vi "setStopServerOcc.vi"(8 "error in (no error)":errorcluster, 11 "TcpServerCmd in":refnum<class "TcpServerCmd.lvclass">) -> (0 "error out":errorcluster, 3 "TcpServerCmd out":refnum<class "TcpServerCmd.lvclass">)   [LabVIEW 2018, in "TcpServerCmd.lvclass"]
doc: "Set the stopServer occurrence to stop the runServer.vi."
uses:
  TcpServerCmd.lvclass
  home/pcortes/github/ts_labview_tcp_json/src/TcpServerBase/TcpServerBase.lvclass
  TcpServerBase/TcpServerBase.lvclass/TcpServerBase.ctl
  TcpServerBase/TcpServerBase.lvclass
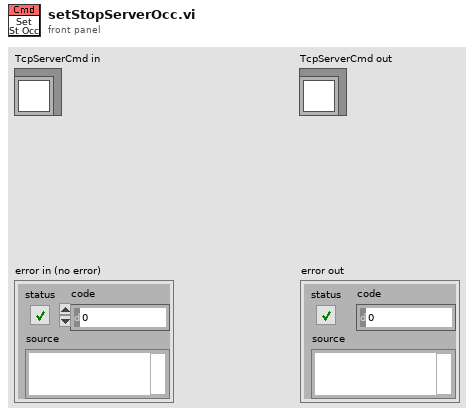
[diagram p1: front panel]
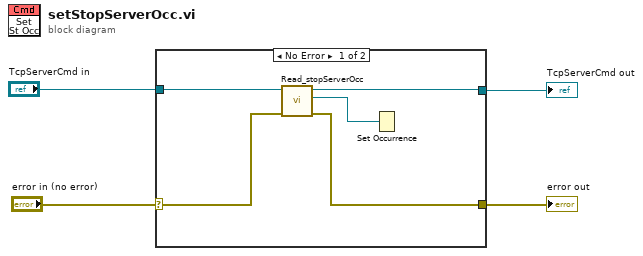
[diagram p0: block diagram]
diagram:
  n1 = case shown="No Error" "error in (no error)" {
    selector: "error in (no error)" -> [w7 w11]
    tunnel: "TcpServerCmd in" -> [w8 w10]
    tunnel: [w6 w11] -> w2
    tunnel: [w5 w10] -> w1
    frame No Error {
      n2 = call "Read_stopServerOcc.vi"("error in (no error)"=w7, "TcpServerBase in"=w8) -> ("error out"=w6:errorcluster, "stopServerOcc"=w9:refnum<k4>, "TcpServerBase out"=w5:refnum<class "TcpServerCmd.lvclass">)  [unwired: 7 in]
      n3 = Set Occurrence(w9) -> ()
    }
    frame Error {
    }
  }
  "error out" <- w2
  "TcpServerCmd out" <- w1
